vi "Write_to_log_file.vi"(6 "User added comment":string, 8 "End time":dbl format="%.2f", 9 "Start time":dbl format="%.2f", 11 "Folder/file":path) -> (0 "File Updated?":bool)   [LabVIEW 2022 SP3]
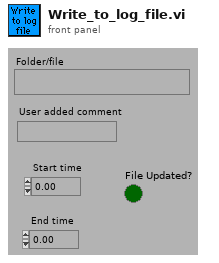
[diagram p1: front panel]
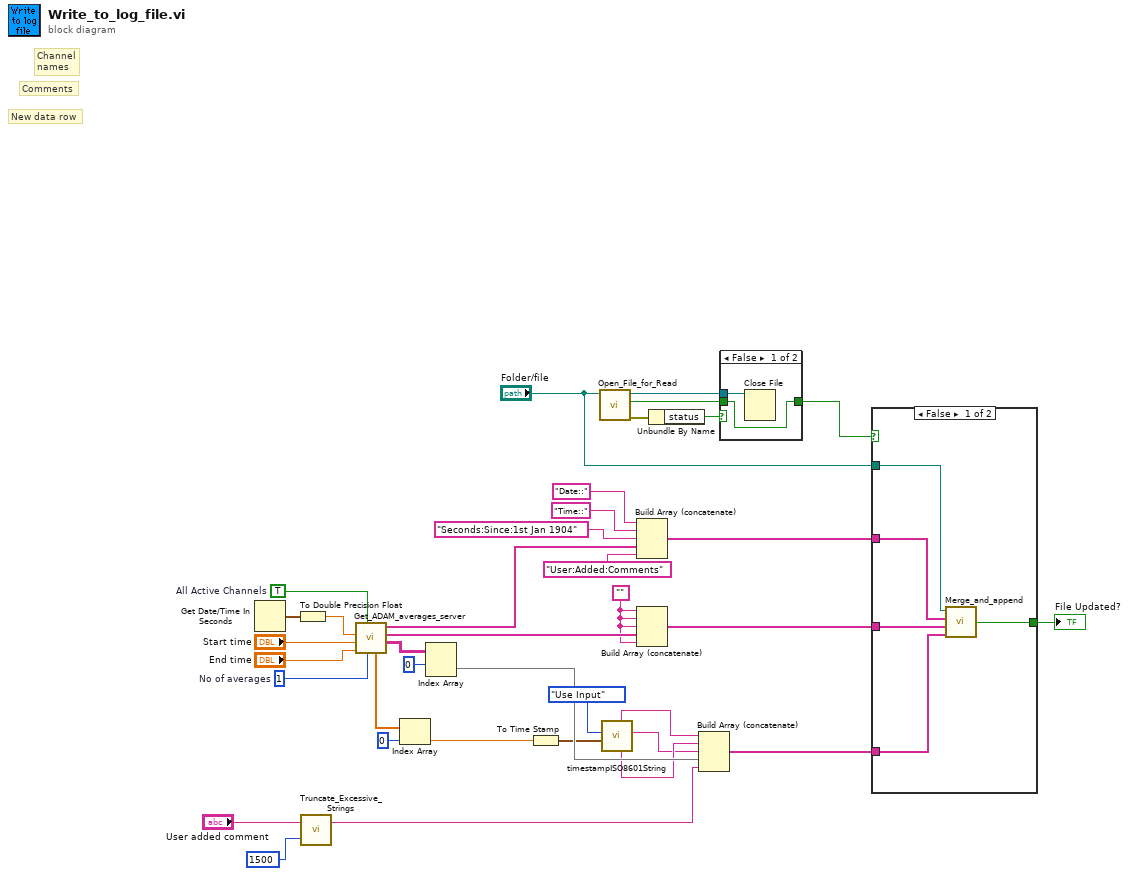
[diagram p0: block diagram]
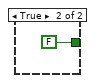
[diagram p2: hidden frame]
diagram:
  w1 = ""
  w27 = 1  # No of averages
  w31 = TRUE  # All Active Channels
  # "Comments"
  # "New data row"
  # "Channel\nnames"
  n1 = Get Date/Time In Seconds() -> (seconds since 1Jan1904=w22:timestamp)
  n2 = To Double Precision Float(number=w22) -> (double precision float=w30:dbl)
  n3 = call "Truncate_Excessive_Strings.vi"("Max String Length"=1500, "String"="User added comment") -> ("Truncated String"=w16:string)  [unwired: 1 in]
  n4 = call "Get_ADAM_averages_server.vi"("No of averages"=w27, "All Active Channels"=w31, "End time"="End time", "Start time"="Start time", "Clients time"=w30) -> ("Values"=w23:string[][], "Comments"=w37:string[], "Titles"=w36:string[], "Times"=w25:dbl[])  [unwired: 1 in, 1 out]
  n5 = Index Array(array=w25, index=0 ("Index")) -> (element=w5:dbl)
  n6 = Index Array(array=w23, index (row)=0) -> (element=w35:string[])  [unwired: 1 in]
  n7 = To Time Stamp(1:w5) -> (0:w7:timestamp)
  n8 = call "Open_File_for_Read.vi"("file path"="Folder/file") -> ("error out"=w14:errorcluster, "Permission error?"=w10:bool, "refnum"=w12:refnum<file>)  [unwired: 8 out]
  n9 = call "timestampISO8601String.vi"("Time Stamp"=w7, "When?"=enum16{"Now", "Use Input"}."Use Input") -> ("timestampString"=w2:string, "Time(24h)"=w3:string, "Date(YYYY-MM-DD)"=w4:string)  [unwired: 4 in, 3 out]
  n10 = Build Array (concatenate)("Date::", "Time::", "Seconds:Since:1st Jan 1904", w36, "User:Added:Comments") -> (w34:string[])
  n11 = Build Array (concatenate)(w1, w1, w1, w37, w1) -> (w32:string[])
  n12 = Unbundle By Name(w14) -> ("status"=w13:bool)
  n13 = Build Array (concatenate)(w4, w3, w2, w35, w16) -> (w33:string[])
  n14 = case shown="False" w13 {
    tunnel: w12 -> [w39 _]
    tunnel: [w38 w40] -> w9
    tunnel: w10 -> [w38 w40]
    frame False {
      n15 = Close File(refnum=w39) -> ()  [unwired: 1 in, 2 out]
    }
    frame True {
    }
  }
  n16 = case shown="False" w9 {
    tunnel: w34 -> [w45 _]
    tunnel: w32 -> [w44 _]
    tunnel: w33 -> [w43 _]
    tunnel: [w42 FALSE ("File Updated?")] -> w15
    tunnel: "Folder/file" -> [w41 _]
    frame False {
      n17 = call "Merge_and_append.vi"("New Row"=w43, "Comments"=w44, "Channel Names"=w45, "Path name"=w41) -> ("File Updated?"=w42:bool)
    }
    frame True {
    }
  }
  "File Updated?" <- w15
